vi "WebCam.DLGVideoSource.vi"(0 "Handle":i32, 11 "ErrorIn":errorcluster) -> (4 "HandleOut":i32, 15 "ErrorOut":errorcluster)   [LabVIEW 2021]
uses:
  User32.WebCam_WM_Events.ctl
  User32.SendMessageA_num.vi
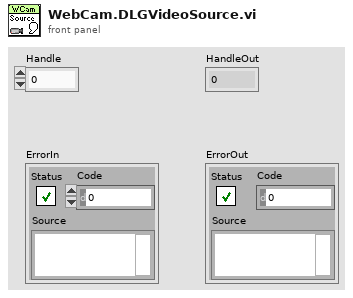
[diagram p1: front panel]
types:
  T1 = typedef "User32.WebCam_WM_Events.ctl" = i32
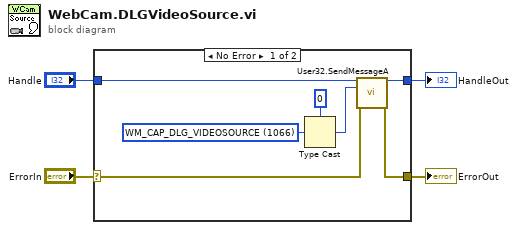
[diagram p0: block diagram]
diagram:
  n1 = case shown="No Error" "ErrorIn" {
    selector: "ErrorIn" -> [w10 w13]
    tunnel: "Handle" -> [w6 w12]
    tunnel: [w5 w12] -> w1
    tunnel: [w11 w13] -> w4
    frame No Error {
      w8 = T1 1066 items=["WM_CAP_DRIVER_CONNECT"=1034, "WM_CAP_DRIVER_DISCONNECT"=1035, "WM_CAP_DRIVER_GET_NAME"=1036, "WM_CAP_DRIVER_GET_VERSION"=1037, "WM_CAP_DRIVER_GET_CAPS"=1038, "WM_CAP_EDIT_COPY"=1054, "WM_CAP_SEQUENCE"=1086, "WM_CAP_FILE_SAVEAS"=1047, "WM_CAP_SET_SCALE"=1077, "WM_CAP_SET_PREVIEWRATE"=1076, "WM_CAP_SET_PREVIEW"=1074, "WM_CAP_SET_OVERLAY"=1075, "WM_CAP_FILE_SAVEDIB"=1049, "WM_CAP_SET_MCI_DEVICE"=1090, "WM_CAP_GET_MCI_DEVICE"=1091, "WM_CAP_DLG_VIDEOSOURCE"=1066] ("Ring")
      n2 = Type Cast(type=0 ("wParam"), x=w8) -> (*(type *) &x=w9:i32)
      n3 = call-poly "User32.SendMessageA.vi"("HWnd"=w6, "Msg"=w9, "ErrorIn"=w10) -> ("HWndOut"=w5:i32, "ErrorOut"=w11:errorcluster)  [unwired: 11 in]
    }
    frame Error {
    }
  }
  "ErrorOut" <- w4
  "HandleOut" <- w1
